vi "Simple UDP - Sender.vi"(9 "Data":dbl[](array[numeric])) -> ()   [LabVIEW 2016]
doc: "The UDP protocol differs from TCP in that there is no error-checking with the packets of information that are sent, and thus no guarantee whatsoever that an intended recipient will actually receive a given piece of data.\n\nUDP does offer the ability to \"broadcast\" data across a network--simply specify an IP Address of all ones (255.255.255.255) to attempt to broadcast information network-wide. Keep in mind that routers and other network hardware will generally refuse to forward the broadcast beyond certain points, so the extent of the broadcast will in practice be limited."
panel:
  in  "Stop":bool
  # "Overview: Demonstrates the use of the UDP functions to send data over a UDP connection.\nInstructions:\n1. Run the VI.\n2. Open Simple UDP - Receiver.vi and follow the instructions on its front panel.\n3. Click Stop to stop the VI."
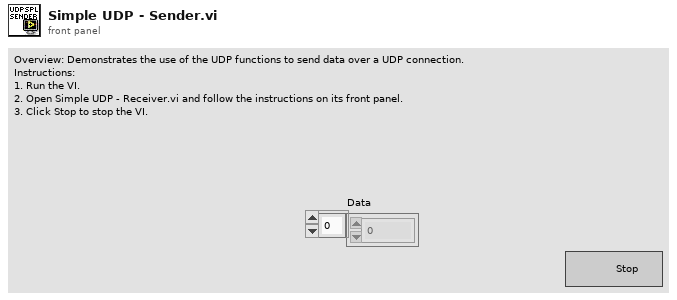
[diagram p1: front panel]
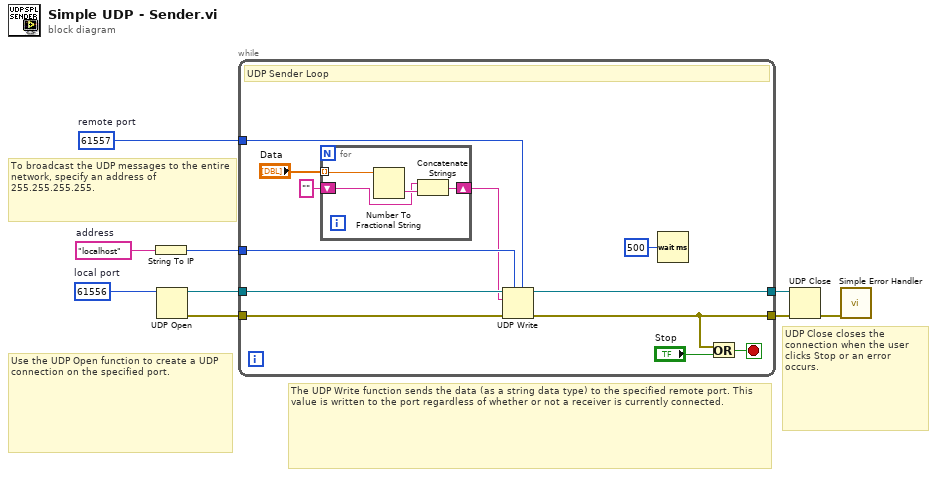
[diagram p0: block diagram]
diagram:
  w1 = u16 61557  # remote port
  w2 = u16 61556  # local port
  w7 = "localhost"  # address
  # "To broadcast the UDP messages to the entire network, specify an address of 255.255.255.255."
  # "UDP Close closes the connection when the user clicks Stop or an error occurs."
  # "The UDP Write function sends the data (as a string data type) to the specified remote port. This value is written to the port regardless of whether or not a receiver is currently connected."
  # "Use the UDP Open function to create a UDP connection on the specified port."
  n1 = String To IP(1:w7) -> (0:w5:u32)
  n2 = UDP Open(11:w2) -> (port=w4:refnum<k16>, 0:w3:errorcluster)  [unwired: 4 in, 1 out]
  n3 = while {
    tunnel: [w16] -> w8
    tunnel: w4 -> [w21]
    tunnel: w3 -> [w20]
    tunnel: [w17] -> w9
    tunnel: w5 -> [w15]
    tunnel: w1 -> [w13]
    stop <- w19 stop-if-true
    # "UDP Sender Loop"
    n4 = for {
      shift-right: [w24] -> w11
      shift-left: "" -> [w23]
      tunnel: "Data" -> [w22] mode=indexing
      n5 = Number To Fractional String(number=w22) -> (F-format string=w25:string)  [unwired: 3 in]
      n6 = Concatenate Strings(w23, w25) -> (w24:string)
    }
    n7 = UDP Write(address=w15, port or service name=w13, connection ID=w21, data in=w11, 8:w20) -> (error out=w16:errorcluster, 3:w17:refnum<k16>)  [unwired: 1 in]
    n8 = Wait (ms)(milliseconds to wait=u32 500) -> ()  [unwired: 1 out]
    n9 = Or(x=w16, y="Stop") -> (x .or. y?=w19:bool)
  }
  n10 = UDP Close(connection ID=w9, 8:w8) -> (error out=w6:errorcluster)  [unwired: 1 out]
  n11 = call <vilib>:"Simple Error Handler.vi"("error in (no error)"=w6) -> ()  [unwired: 4 in, 5 out]
